vi "RSNRPZ Configure Internal.vi"(7 "Trigger Slope (0: Positive)":i32(ring) items=["Positive", "Negative"], 8 "error in (no error)":errorcluster, 9 "Trigger Level (1.0e-6 W)":dbl=1e-06 format="%.2p", 10 "Channel (1)":i32=1, 11 "VISA session":refnum<visa-resource-name> caption="VISA resource name") -> (0 "error out":errorcluster, 3 "dup VISA session":refnum<visa-resource-name> caption="VISA resource name")   [LabVIEW 2010]
doc: "This VI configures the parameters of internal trigger system.\n\nRemote-control command(s):\nTRIG:DEL:AUTO ON\nTRIG:ATR OFF\nTRIG:COUN 1\nTRIG:DEL 0.0\nTRIG:HOLD 0.0\nTRIG:HYST 3DB\nTRIG:LEV <value>\nTRIG:SLOP POS | NEG\nTRIG:SOUR INT"
uses:
  rsnrpz_32.dll
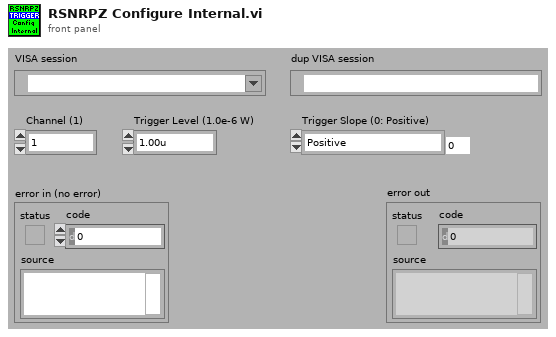
[diagram p1: front panel]
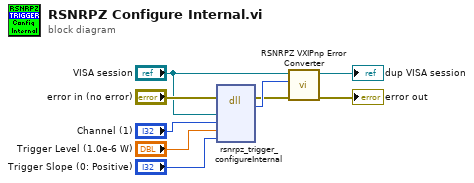
[diagram p0: block diagram]
diagram:
  n1 = dll-call lib="rsnrpz_32.dll" fn="rsnrpz_trigger_configureInternal"(error in="error in (no error)", "VISA Session"="VISA session", "Channel"="Channel (1)", "Trigger Level"="Trigger Level (1.0e-6 W)", "Trigger Slope"="Trigger Slope (0: Positive)") -> (error out=w5:errorcluster, "Status"=w9:i32)  [unwired: 6 in, 1 out]
  n2 = call <instrlib>:"RSNRPZ VXIPnp Error Converter.vi"("error in"=w5, "VXIPnp error code"=w9, "VISA session"="VISA session") -> ("error out"=→"error out":errorcluster, "dup VISA session"=→"dup VISA session":refnum<visa-resource-name>)  [unwired: 7 in]
